vi "Auto Manual selector for shifting.vi"(8 "From Shift":bool, 9 "High Gear button":bool, 10 "Low Gear button":bool, 11 "Manual?":bool) -> (0 "Manually controlled":bool, 1 "High Gear?":bool)   [LabVIEW 2013]
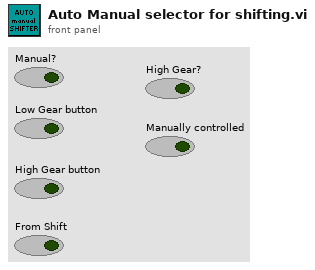
[diagram p1: front panel]
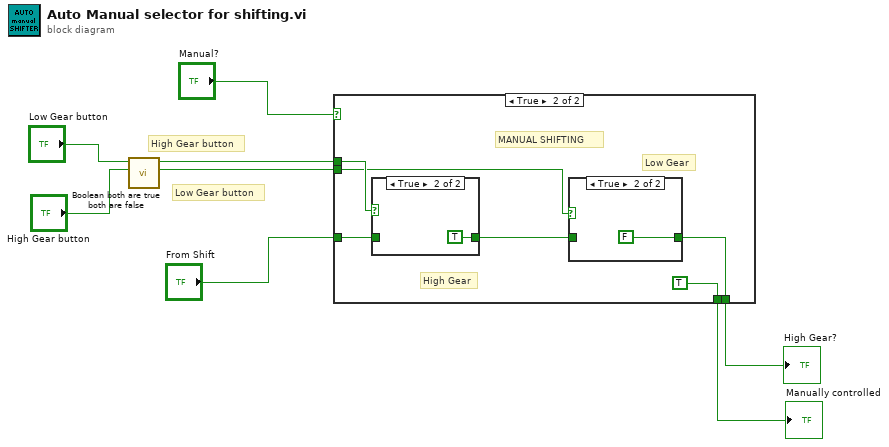
[diagram p0: block diagram]
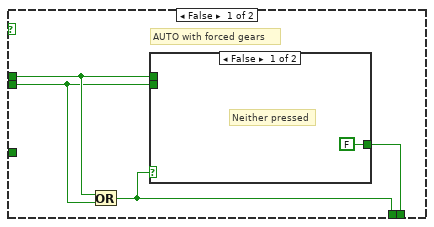
[diagram p2: hidden frame]
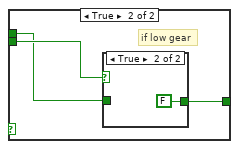
[diagram p3: hidden frame]
diagram:
  # "Low Gear button"
  # "High Gear button"
  n1 = call "Boolean both are true both are false.vi"("Input A"="High Gear button", "Input B"="Low Gear button") -> ("output B"=w5:bool, "output A"=w4:bool)  [unwired: 8 in]
  n2 = case shown="True" "Manual?" {
    tunnel: "From Shift" -> [_ w24]
    tunnel: w4 -> [w11 w22]
    tunnel: w5 -> [w10 w21]
    tunnel: [w12 TRUE] -> w6
    tunnel: [w9 w19] -> w7
    frame False {
      # "AUTO with forced gears"
      n3 = Or(x=w11, y=w10) -> (x .or. y?=w12:bool)
      n4 = case shown="False" w12 {
        tunnel: w11 -> [_ w15]
        tunnel: w10 -> [_ w16]
        tunnel: [FALSE ("output A") w14] -> w9
        frame False {
          # "Neither pressed"
        }
        frame True {
          # "if low gear"
          n5 = case shown="True" w16 {
            tunnel: w15 -> [w17 _]
            tunnel: [w17 FALSE ("output A")] -> w14
            frame False {
            }
            frame True {
            }
          }
        }
      }
    }
    frame True {
      # "High Gear"
      # "Low Gear"
      # "MANUAL SHIFTING"
      n6 = case shown="True" w22 {
        tunnel: w24 -> [w25 _]
        tunnel: [w25 TRUE ("be in high gear?")] -> w23
        frame False {
        }
        frame True {
        }
      }
      n7 = case shown="True" w21 {
        tunnel: w23 -> [w27 _]
        tunnel: [w27 FALSE ("be in high gear?")] -> w19
        frame False {
        }
        frame True {
        }
      }
    }
  }
  "High Gear?" <- w7
  "Manually controlled" <- w6
